vi "Set VI Run On Open Property.vi"(8 "error in (no error)":errorcluster, 10 "Run When Opened?":bool, 11 "VI Path":path) -> (0 "error out":errorcluster)   [LabVIEW 2016, in "SLL Scripting.lvlib"]
doc: "Set/Unset the VI's Run On Open Property"
uses:
  SLL Scripting.lvlib
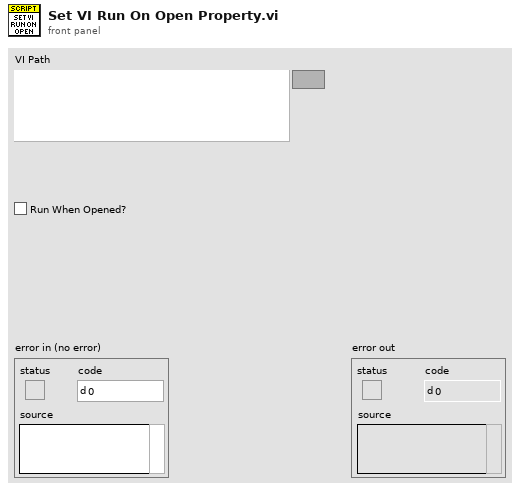
[diagram p1: front panel]
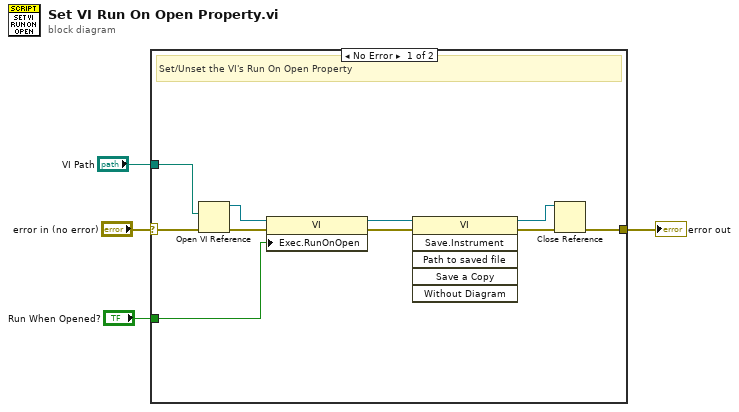
[diagram p0: block diagram]
diagram:
  n1 = case shown="No Error" "error in (no error)" {
    selector: "error in (no error)" -> [w14 w15]
    tunnel: [w6 w15] -> w3
    tunnel: "VI Path" -> [w12 _]
    tunnel: "Run When Opened?" -> [w9 _]
    frame No Error {
      # "Set/Unset the VI's Run On Open Property"
      n2 = Open VI Reference(vi path=w12, error in (no error)=w14) -> (vi reference=w10:refnum<vi>, error out=w13:errorcluster)  [unwired: 4 in]
      n3 = property class="VI"(reference=w10, error in=w13, "Exec.RunOnOpen"=w9) -> (reference out=w7:refnum<vi>, error out=w11:errorcluster)
      n4 = invoke class="VI" method="Save.Instrument"(reference=w7, error in=w11) -> (reference out=w5:refnum<vi>, error out=w8:errorcluster)  [unwired: 4 in, 4 out]
      n5 = Close Reference(reference=w5, error in (no error)=w8) -> (error out=w6:errorcluster)
    }
    frame Error {
    }
  }
  "error out" <- w3
